vi "calculate tiff files size.vi"() -> (3 "no. of channels":i16)   [LabVIEW 2017]
doc: "SciScan 1.2 160622"
uses:
  Custom Controls/file format type def.ctl
  GFG/GFGnumericGet.vi
  GFG/GFGfpRefGet.vi
  GFG/GFG library.lvlib
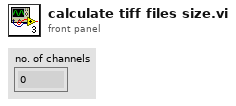
[diagram p1: front panel]
types:
  T1 = typedef "file format type def.ctl" = enum16{"16bit raw", "32bit raw", "16bit multi-tiff (interleave)", "16bit multi-tiff (separate)", "16bit multi-tiff (stacked)", "32bit multi-tiff (interleave)", "32bit multi-tiff (separate)", "32bit multi-tiff (stacked)", "16bit tiff series (interleave)", "16bit tiff series (separate)", "16bit tiff series (stacked)", "32bit tiff series (interleave)", "32bit tiff series (separate)", "32bit tiff series (stacked)"}
  T2 = enum8{"Enabled", "Disabled", "Disabled and Grayed Out"}
  T3 = cluster{"WaveformChartRef":refnum<vi>, "DigitalRef":refnum<vi>, "ArrayRef":refnum<vi>, "TabControlRef":refnum<vi>, "EnumRef":refnum<vi>, "RingRef":refnum<vi>, "BooleanRef":refnum<vi>, "KnobRef":refnum<vi>, "SlideRef":refnum<vi>, "PathRef":refnum<vi>, "StringRef":refnum<vi>, "ComboBox":refnum<vi>, "WaveformGraphRef":refnum<vi>}
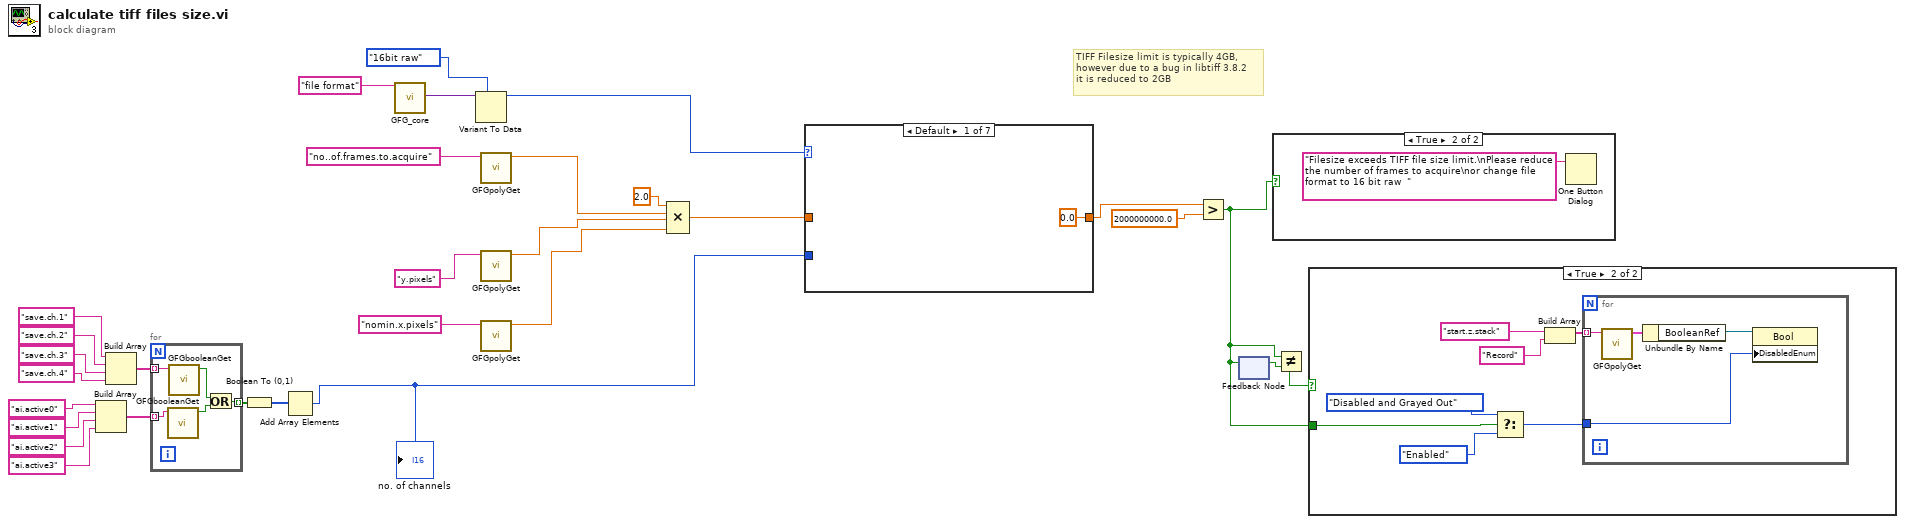
[diagram p0: block diagram]
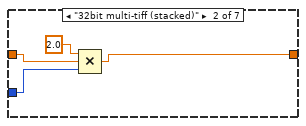
[diagram p4: hidden frame]
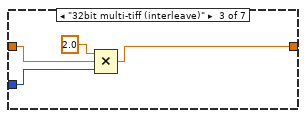
[diagram p5: hidden frame]
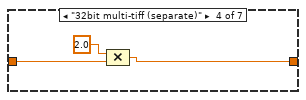
[diagram p6: hidden frame]
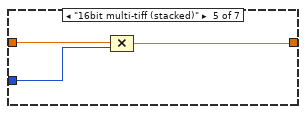
[diagram p7: hidden frame]
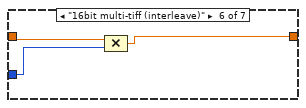
[diagram p8: hidden frame]
diagram:
  # "TIFF Filesize limit is typically 4GB,\nhowever due to a bug in libtiff 3.8.2\nit is reduced to 2GB"
  n1 = Build Array("ai.active0" ("Variable Name in"), "ai.active1" ("Variable Name in"), "ai.active2" ("Variable Name in"), "ai.active3" ("Variable Name in")) -> (w21:string[])
  n2 = Build Array("save.ch.1" ("Variable Name in"), "save.ch.2" ("Variable Name in"), "save.ch.3" ("Variable Name in"), "save.ch.4" ("Variable Name in")) -> (w16:string[])
  n3 = for {
    tunnel: w16 -> [w35] mode=indexing
    tunnel: w21 -> [w34] mode=indexing
    tunnel: [w31] -> w11 mode=indexing
    n4 = call "GFGbooleanGet.vi"("Variable Name in"=w34) -> ("Boolean Value OUT"=w33:bool)  [unwired: 9 in, 1 out]
    n5 = call "GFGbooleanGet.vi"("Variable Name in"=w35) -> ("Boolean Value OUT"=w32:bool)  [unwired: 9 in, 1 out]
    n6 = Or(x=w32, y=w33) -> (x .or. y?=w31:bool)
  }
  n7 = Boolean To (0,1)(Boolean=w11) -> (0, 1=w10:i16[])
  n8 = Add Array Elements(numeric array=w10) -> (sum=w6:i16)
  "no. of channels" <- w6
  n9 = call "GFG_core.vi"("Variable Name in"="file format") -> ("Variant Out"=w29:variant)  [unwired: 12 in, 6 out]
  n10 = Variant To Data(type=file_format_type_def."16bit raw" ("file format"), Variant=w29) -> (data=w8:T1)  [unwired: 1 in, 1 out]
  n11 = call-poly "GFGpolyGet.vi"("Variable Name in"="no..of.frames.to.acquire") -> ("Numeric"=w24:dbl)  [unwired: 8 in, 2 out]
  n12 = call-poly "GFGpolyGet.vi"("Variable Name in"="y.pixels" ("Tag in")) -> ("Numeric"=w22:dbl)  [unwired: 8 in, 2 out]
  n13 = call-poly "GFGpolyGet.vi"("Variable Name in"="nomin.x.pixels" ("Tag in")) -> ("Numeric"=w23:dbl)  [unwired: 8 in, 2 out]
  n14 = Compound Arithmetic op=MULTIPLY(2.0 ("value"), w24, w22, w23) -> (w7:dbl)
  n15 = case shown="Default" w8 {
    tunnel: w7 -> [_ w38 w43 w46 w50 w53 w54]
    tunnel: w6 -> [_ w39 w42 _ w49 w52 _]
    tunnel: [0.0 w37 w41 w45 w48 w51 w54] -> w4
    frame Default {
    }
    frame "32bit multi-tiff (stacked)" {
      n16 = Compound Arithmetic op=MULTIPLY(2.0 ("value"), w38, w39) -> (w37:dbl)
    }
    frame "32bit multi-tiff (interleave)" {
      n17 = Compound Arithmetic op=MULTIPLY(2.0 ("value"), w43, w42) -> (w41:dbl)
    }
    frame "32bit multi-tiff (separate)" {
      n18 = Compound Arithmetic op=MULTIPLY(2.0 ("value"), w46) -> (w45:dbl)
    }
    frame "16bit multi-tiff (stacked)" {
      n19 = Compound Arithmetic op=MULTIPLY(w50, w49) -> (w48:dbl)
    }
    frame "16bit multi-tiff (interleave)" {
      n20 = Compound Arithmetic op=MULTIPLY(w53, w52) -> (w51:dbl)
    }
    frame "16bit multi-tiff (separate)" {
    }
  }
  n21 = Greater?(x=w4, y=2000000000.0 ("result")) -> (0:w3:bool)
  n22 = feedback-in #1(w3) -> ()
  n23 = feedback #1() -> (w1:bool)  [unwired: 1 in]
  n24 = case shown="True" w3 {
    frame False {
    }
    frame True {
      n25 = One Button Dialog(message="Filesize exceeds TIFF file size limit.\nPlease reduce the number of frames to acquire\nor change file format to 16 bit raw  ") -> ()  [unwired: 1 in, 1 out]
    }
  }
  n26 = Not Equal?(x=w3, y=w1) -> (x != y?=w2:bool)
  n27 = case shown="True" w2 {
    tunnel: w3 -> [_ w56]
    frame False {
    }
    frame True {
      n28 = Select(t=T2."Disabled and Grayed Out" ("Disabled"), s=w56, f=T2."Enabled" ("Disabled")) -> (s? t:f=w59:T2)
      n29 = Build Array("start.z.stack" ("Variable Name in"), "Record" ("Variable Name in")) -> (w58:string[])
      n30 = for {
        tunnel: w59 -> [w64]
        tunnel: w58 -> [w63] mode=indexing
        n31 = call-poly "GFGpolyGet.vi"("Variable Name in"=w63) -> ("output cluster"=w66:T3)  [unwired: 9 in, 1 out]
        n32 = Unbundle By Name(w66) -> ("BooleanRef"=w65:refnum<vi>)
        n33 = property class="Bool"(reference=w65, "DisabledEnum"=w64) -> ()  [unwired: 1 in, 2 out]
      }
    }
  }
